vi "test_image_resize.vi"   [LabVIEW 2011]
uses:
  <vilib>/vision/NI_Vision_Development_Module.lvlib
types:
  T1 = typedef "Image Type" = u32
  T2 = typedef "IMAQ Image.ctl" = refnum<image>
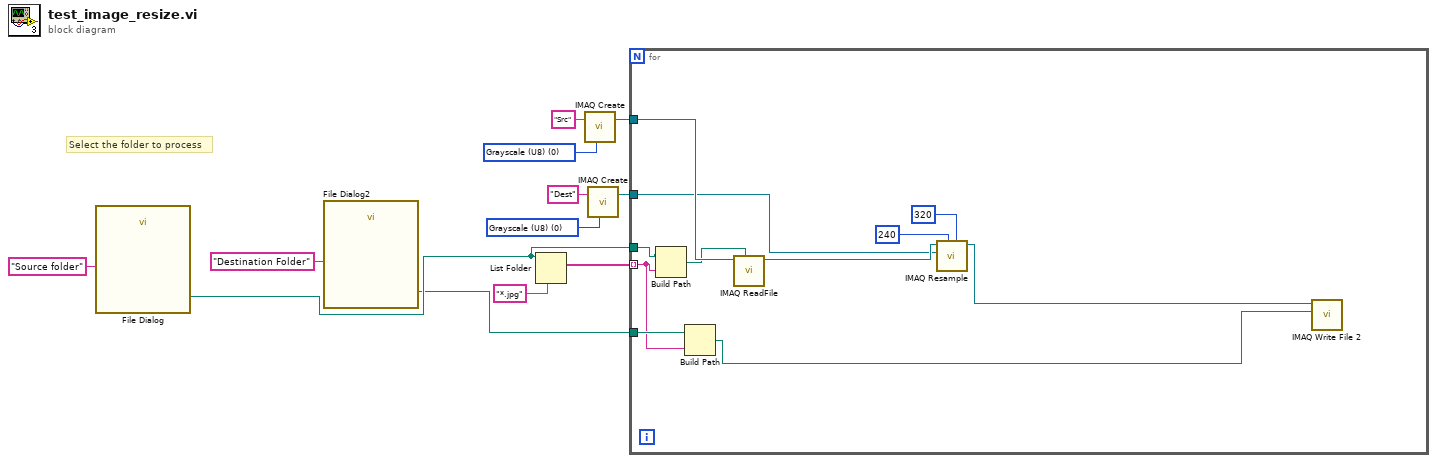
[diagram p0: block diagram]
diagram:
  w5 = T1 0 items=["Grayscale (U8)", "Grayscale (I16)", "Grayscale (SGL)", "Complex (CSG)", "RGB (U32)", "HSL (U32)", "RGB (U64)", "Grayscale (U16)"] ("Image Type")
  w7 = T1 0 items=["Grayscale (U8)", "Grayscale (I16)", "Grayscale (SGL)", "Complex (CSG)", "RGB (U32)", "HSL (U32)", "RGB (U64)", "Grayscale (U16)"] ("Image Type")
  # "Select the folder to process"
  n1 = call "File Dialog"("prompt"="Source folder") -> ("selected path"=w3:path)  [unwired: 11 in, 3 out]
  n2 = call "File Dialog2"("prompt"="Destination Folder") -> ("selected path"=w1:path)  [unwired: 11 in, 3 out]
  n3 = List Folder(path=w3, pattern="*.jpg") -> (filenames=w9:string[])  [unwired: 2 in, 3 out]
  n4 = call "IMAQ Create"("Image Name"="Src", "Image Type"=w7) -> ("New Image"=w4:T2)  [unwired: 3 in, 1 out]
  n5 = call "IMAQ Create"("Image Name"="Dest", "Image Type"=w5) -> ("New Image"=w2:T2)  [unwired: 3 in, 1 out]
  n6 = for {
    tunnel: w9 -> [w19] mode=indexing
    tunnel: w4 -> [w23]
    tunnel: w3 -> [w21]
    tunnel: w2 -> [w16]
    tunnel: w1 -> [w20]
    n7 = Build Path(base path=w21, name or relative path=w19) -> (appended path=w22:path)
    n8 = Build Path(base path=w20, name or relative path=w19) -> (appended path=w18:path)
    n9 = call "IMAQ ReadFile"("File Path"=w22, "Image"=w23) -> ("Image Out"=w17:T2)  [unwired: 5 in, 4 out]
    n10 = call "IMAQ Resample"("X Resolution"=320, "Y Resolution"=240, "Image Dst"=w16, "Image Src"=w17) -> ("Image Dst Out"=w15:T2)  [unwired: 6 in, 1 out]
    n11 = call-poly "IMAQ Write File 2"("File Path"=w18, "Image"=w15) -> ()  [unwired: 8 in, 2 out]
  }
